vi "Adjust Magnetic Field_Continuous CW.vi"() -> ()   [LabVIEW 2020]
uses:
  Labview Library/Libraries/UT_Utilities/Utilities.lvlib
  Labview Library/Libraries/UT_Utilities/Support/Peak Parameter.ctl
  Labview Library/Libraries/Basic Experiment/Basic Experiment.lvlib
  Labview Library/Libraries/UT_Utilities/Support/Lorentizan Fit Parameter.ctl
  Labview Library/Libraries/Basic Experiment/CW settings.ctl
panel:
  in  "PS":string="X20.2 Y-0.4 Z16.5"
  in  "Theory Right Peak":dbl=1374.5
  in  "Calculate Right Peak":bool
  in  "Theory Left Peak":dbl=1374.5
  in  "Calculate Left Peak":bool
  in  "Add History":bool=TRUE
  in  "History":T2(array[cluster])
  in  "Zero Field Frequency":dbl=1360.0
  in  "Left Peak Settings":T3={"Num Pts"=20, "Start freq"=1205.0, "Stop freq"=1125.0, " dBm"=-10.0, "Loop times"=30000, "Ratio Thre(abs)"=0.03, "AutoTrace Before Exp"=FALSE, "RepoSave"=FALSE, "Peak Num Limit "=1}
  out "CW Left":cluster{"x":dbl[], "y":dbl[]}[](graph)=[{"x"=[1205.0, 1201.0, 1197.0, 1193.0, 1189.0, 1185.0, 1181.0, 1177.0, 1173.0, 1169.0, 1165.0, 1161.0, 1157.0, 1153.0, 1149.0, 1145.0, 1141.0, 1137.0, 1133.0, 1129.0, 1125.0], "y"=[-0.011159938681655596, -0.025153553670663936, -0.011876586772236327, 0.00021785543113589823, -0.012618639098234258, 0.004807904371223149, -0.00332547845045918, -0.001677185858675023, -0.0044172764590398005, -0.010320538540412821, -0.01357328707718994, -0.010368157455408136, -0.011699885854772149, -0.02274875266501088, -0.007152347209920283, -0.012399964822794828, -0.007602415395977236, -0.012597193866469744, -0.01720978929459495, -0.014711782800588472, -0.015376683926209849]}, {"x"=array[301 elements], "y"=[nan, nan, nan, nan, nan, nan, nan, nan, nan, nan, nan, nan, nan, nan, nan, nan, nan, nan, nan, nan, nan, nan, nan, nan, nan, nan, nan, nan, nan, nan, nan, nan, nan, nan, nan, nan, nan, nan, nan, nan, nan, nan, nan, nan, nan, nan, nan, nan, nan, nan, nan, nan, nan, nan, nan, nan, nan, nan, nan, nan, nan, nan, nan, nan, nan, nan, nan, nan, nan, nan, nan, nan, nan, nan, nan, nan, nan, nan, nan, nan, nan, nan, nan, nan, nan, nan, nan, nan, nan, nan, nan, nan, nan, nan, nan, nan, nan, nan, nan, nan, nan, nan, nan, nan, nan, nan, nan, nan, nan, nan, nan, nan, nan, nan, nan, nan, nan, nan, nan, nan, nan, nan, nan, nan, nan, nan, nan, nan, nan, nan, nan, nan, nan, nan, nan, nan, nan, nan, nan, nan, nan, nan, nan, nan, nan, nan, nan, nan, nan, nan, nan, nan, nan, nan, nan, nan, nan, nan, nan, nan, nan, nan, nan, nan, nan, nan, nan, nan, nan, nan, nan, nan, nan, nan, nan, nan, nan, nan, nan, nan, nan, nan, nan, nan, nan, nan, nan, nan, nan, nan, nan, nan, nan, nan, nan, nan, nan, nan, nan, nan, nan, nan, nan, nan, nan, nan, nan, nan, nan, nan, nan, nan, nan, nan, nan, nan, nan, nan, nan, nan, nan, nan, nan, nan, nan, nan, nan, nan, nan, nan, nan, nan, nan, nan, nan, nan, nan, nan, nan, nan, nan, nan, nan, nan, nan, nan, nan, nan, nan, nan, nan, nan, nan, nan, nan, nan, nan, nan, nan, nan, nan, nan, nan, nan, nan, nan, nan, nan, nan, nan, nan, nan, nan, nan, nan, nan, nan, nan, nan, nan, nan, nan, nan, nan, nan, nan, nan, nan, nan, nan, nan, nan, nan, nan, nan, nan, nan, nan, nan, nan, nan]}]
  in  "Left Fit Parameter":T4={"Background"=nan, "Peaks Parameter"=[]}
  in  "Right Fit Parameter":T4={"Background"=0.0056945852649640805, "Peaks Parameter"=[{"Amplitude"=-0.07797747065966305, "Position"=1532.2862299382655, "Width"=14.69533523973655}]}
  out "CW Right":cluster{"x":dbl[], "y":dbl[]}[](graph)=[{"x"=[1520.0, 1523.5, 1527.0, 1530.5, 1534.0, 1537.5, 1541.0, 1544.5, 1548.0, 1551.5, 1555.0, 1558.5, 1562.0, 1565.5, 1569.0, 1572.5, 1576.0, 1579.5, 1583.0, 1586.5, 1590.0], "y"=[-0.04503608389240439, -0.048468161356584064, -0.06917413643541893, -0.06935774109701642, -0.06266092515315635, -0.06993709008164904, -0.057095591522847176, -0.044065051622916525, -0.03324762033653629, -0.026683780314801054, -0.011314460872701045, 0.002465096474912041, -0.0038063202620164647, -0.005934718100890208, 0.0013360945954973612, 0.006420007158196134, -0.005723031875956611, -0.014175914235718875, -0.006224388082844169, 0.008040380578014025, -0.010785893304690297]}, {"x"=array[301 elements], "y"=array[301 elements]}]
  in  "Right Peak Settings":T3={"Num Pts"=20, "Start freq"=1520.0, "Stop freq"=1590.0, " dBm"=-13.0, "Loop times"=30000, "Ratio Thre(abs)"=0.04, "AutoTrace Before Exp"=FALSE, "RepoSave"=FALSE, "Peak Num Limit "=1}
  in  "Left Peak":bool
  in  "Right Peak":bool=TRUE
  in  "stop":bool
  in  "Enqueue Element":bool
  # "CW Settings"
  # "CW Settings"
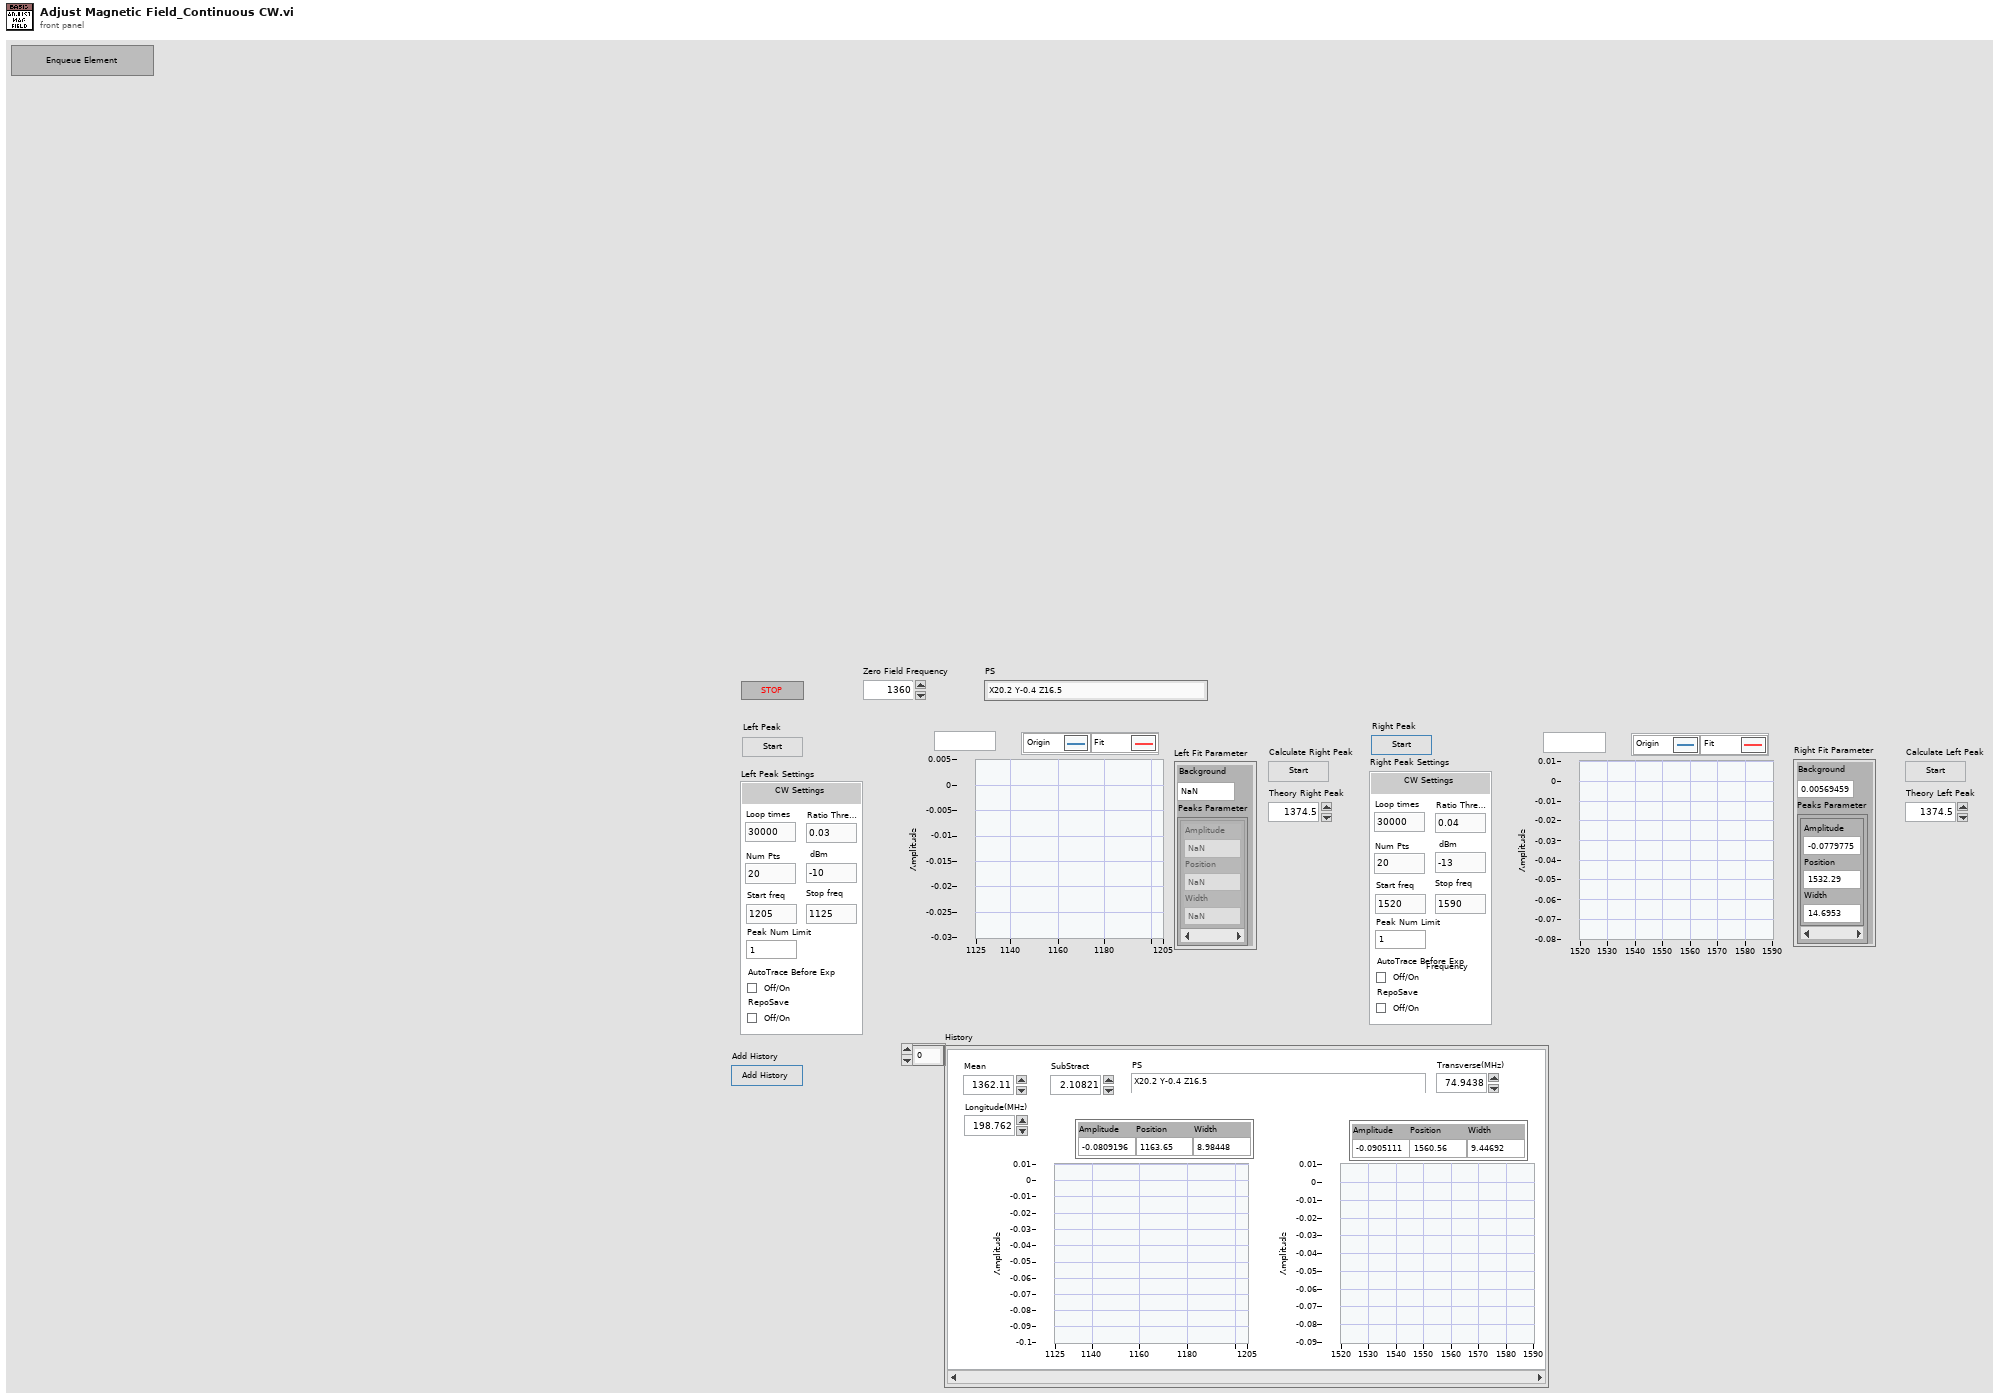
[diagram p1: front panel]
types:
  T1 = typedef "Utilities.lvlib/Peak Parameter.ctl" = cluster{"Amplitude":dbl, "Position":dbl, "Width":dbl}
  T2 = cluster{"Mean":dbl, "SubStract":dbl, "PS":string, "CW Left":cluster{"x":dbl[], "y":dbl[]}[], "CW Right":cluster{"x":dbl[], "y":dbl[]}[], "Left Peak Parameter":T1, "Right Peak Parameter":T1, "Longitude(MHz)":dbl, "Transverse(MHz)":dbl}[]
  T3 = typedef "Basic Experiment.lvlib/CW settings.ctl" = cluster{"Num Pts":i32, "Start freq":dbl, "Stop freq":dbl, " dBm":dbl, "Loop times":i32, "Ratio Thre(abs)":dbl, "AutoTrace Before Exp":bool, "RepoSave":bool, "Peak Num Limit ":i32}
  T4 = typedef "Utilities.lvlib/Lorentizan Fit Parameter.ctl" = cluster{"Background":dbl, "Peaks Parameter":T1[]}
  T5 = cluster{"Mean":dbl, "SubStract":dbl, "PS":string, "CW Left":cluster{"x":dbl[], "y":dbl[]}[], "CW Right":cluster{"x":dbl[], "y":dbl[]}[], "Left Peak Parameter":T1, "Right Peak Parameter":T1, "Longitude(MHz)":dbl, "Transverse(MHz)":dbl}
  T6 = typedef "Basic Experiment.lvlib/CW Results.ctl" = cluster{"Fit Frequency":T7, "Pro":dbl[], "Error Bar":dbl[], "Raw Data Path":path, "Image Path":path}
  T7 = typedef "Basic Experiment.lvlib/CW Fit Frequency.ctl" = cluster{"Fre2":cluster{"Amplitude":dbl, "Position":dbl, "Width":dbl}, "Fre1":cluster{"Amplitude":dbl, "Position":dbl, "Width":dbl}, "Fre3":cluster{"Amplitude":dbl, "Position":dbl, "Width":dbl}, "Background":dbl}
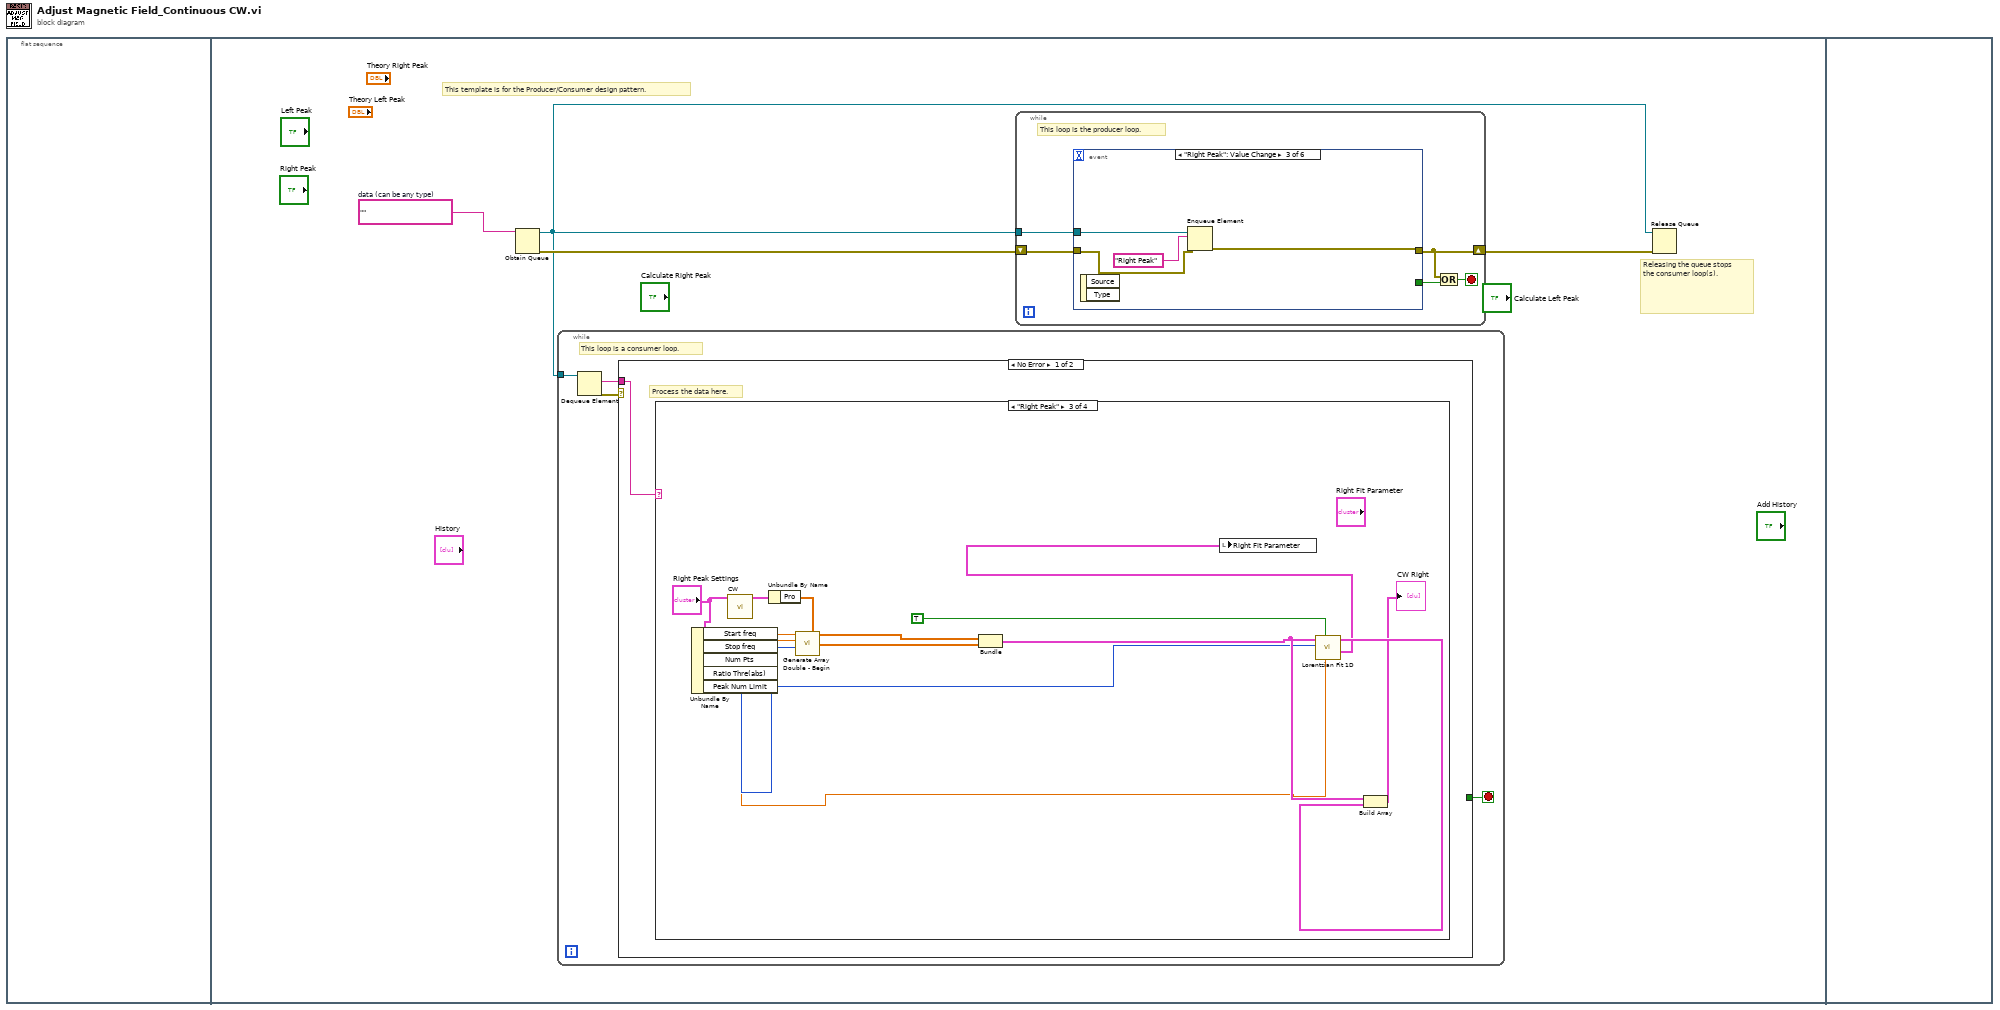
[diagram p0: block diagram]
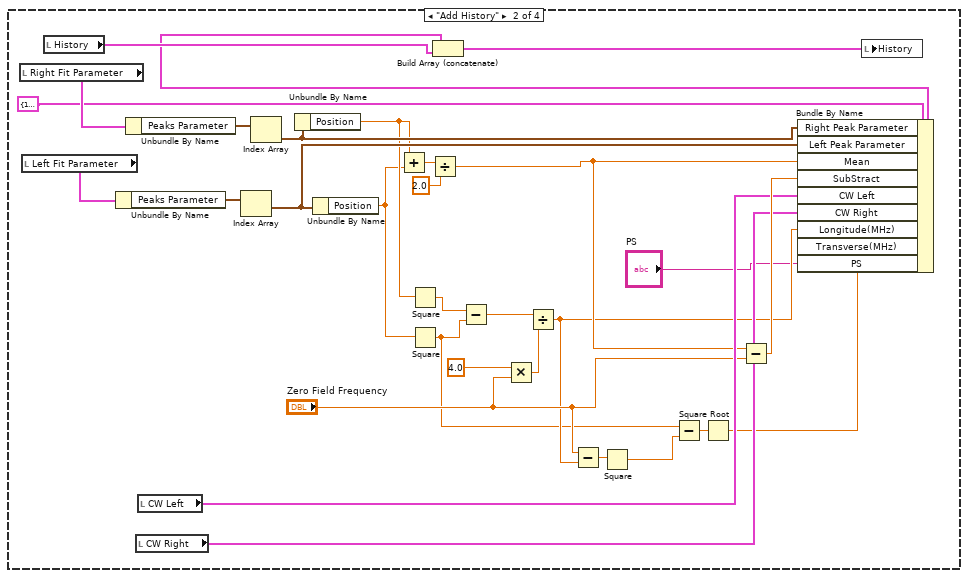
[diagram p3: hidden frame]
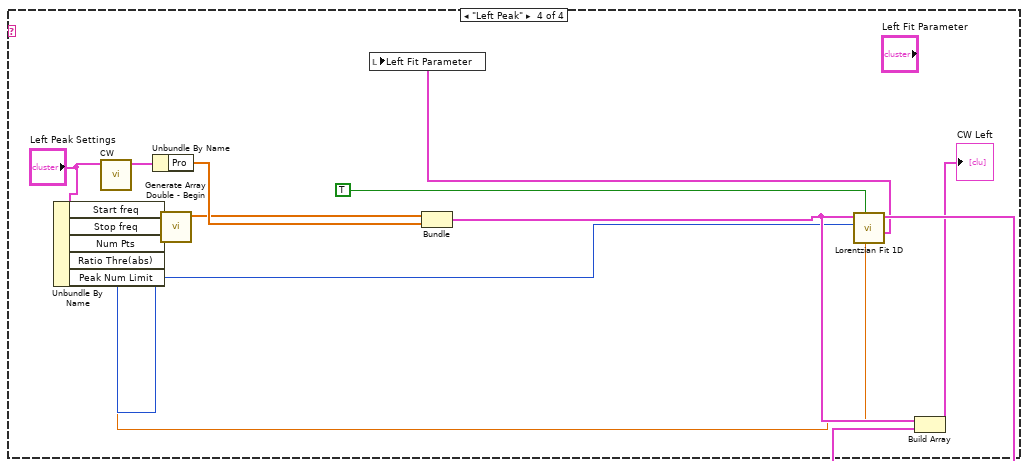
[diagram p4: hidden frame]
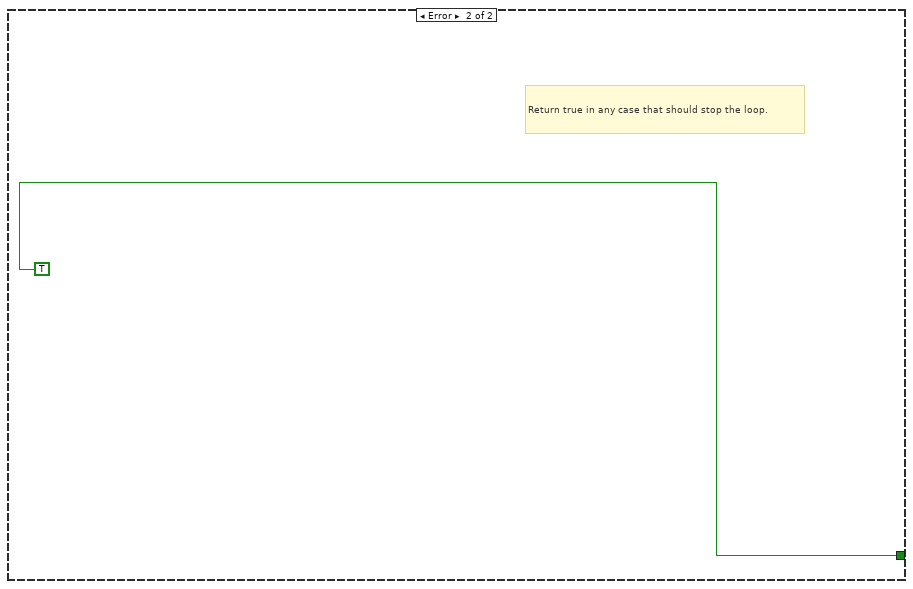
[diagram p5: hidden frame]
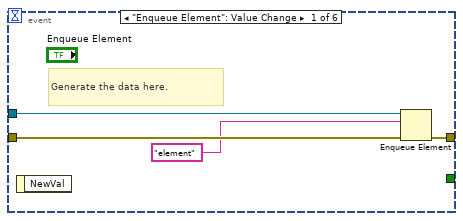
[diagram p6: hidden frame]
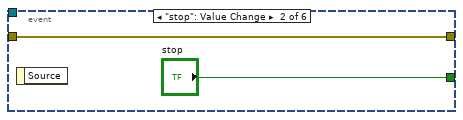
[diagram p7: hidden frame]
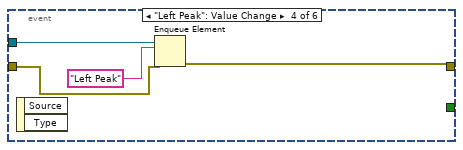
[diagram p8: hidden frame]
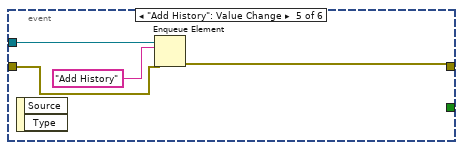
[diagram p9: hidden frame]
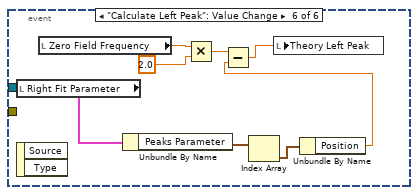
[diagram p10: hidden frame]
diagram:
  n1 = flat-sequence {
    frame #0 {
    }
    frame #1 {
      w2 = ""  # data (can be any type)
      # "Releasing the queue stops the consumer loop(s)."
      # "This template is for the Producer/Consumer design pattern."
      n2 = Obtain Queue(element data type=w2) -> (queue out=w1:refnum<queue>, error out=w4:errorcluster)  [unwired: 4 in, 1 out]
      n3 = while {
        tunnel: w1 -> [w8]
        stop <- w5 stop-if-true
        # "This loop is a consumer loop."
        n4 = Dequeue Element(queue=w8) -> (element=w6:string, error out=w7:errorcluster)  [unwired: 2 in, 2 out]
        n5 = case shown="No Error" w7 {
          tunnel: w6 -> [w9 _]
          tunnel: [_ TRUE] -> w5
          frame No Error {
            # "Process the data here."
            n6 = case shown="\"Right Peak\"" w9 {
              frame "False", Default {
              }
              frame "Add History" {
                n7 = local read "Right Fit Parameter"() -> (w36:T4)
                n8 = local read "Left Fit Parameter"() -> (w39:T4)
                n9 = local read "History"() -> (w31:T2)
                n10 = Unbundle By Name(w39) -> ("Peaks Parameter"=w38:T1[])
                n11 = Unbundle By Name(w36) -> ("Peaks Parameter"=w37:T1[])
                n12 = local read "CW Right"() -> (w28:cluster{"x":dbl[], "y":dbl[]}[])
                n13 = local read "CW Left"() -> (w29:cluster{"x":dbl[], "y":dbl[]}[])
                n14 = Index Array(array=w38) -> (element=w25:T1)  [unwired: 1 in]
                n15 = Index Array(array=w37) -> (element=w24:T1)  [unwired: 1 in]
                n16 = Unbundle By Name(w24) -> ("Position"=w23:dbl)
                n17 = Unbundle By Name(w25) -> ("Position"=w14:dbl)
                n18 = Add(x=w23, y=w14) -> (x+y=w35:dbl)
                n19 = Square(x=w23) -> (x^2=w22:dbl)
                n20 = Square(x=w14) -> (x^2=w11:dbl)
                n21 = Divide(x=w35, y=2.0) -> (x/y=w26:dbl)
                n22 = Subtract(x=w22, y=w11) -> (x-y=w21:dbl)
                n23 = Multiply(x=4.0, y="Zero Field Frequency") -> (x*y=w19:dbl)
                n24 = Divide(x=w21, y=w19) -> (x/y=w17:dbl)
                n25 = Subtract(x="Zero Field Frequency", y=w17) -> (x-y=w16:dbl)
                n26 = Square(x=w16) -> (x^2=w15:dbl)
                n27 = Subtract(x=w11, y=w15) -> (x-y=w13:dbl)
                n28 = Square Root(x=w13) -> (sqrt(x)=w12:dbl)
                n29 = Subtract(x=w26, y="Zero Field Frequency") -> (x-y=w33:dbl)
                n30 = Bundle By Name(cluster=T5 {"Mean"=1414.1094924647537, "SubStract"=39.60949246475366, "PS"="", "CW Left"=[], "CW Right"=[], "Left Peak Parameter"={"Amplitude"=-0.05552543645018247, "Position"=1349.4629709624935, "Width"=6.25}, "Right Peak Parameter"={"Amplitude"=-0.09115089462235382, "Position"=1478.7560139670136, "Width"=6.817754325190208}, "Longitude(MHz)"=nan, "Transverse(MHz)"=nan} ("History"), "Right Peak Parameter"=w24, "Left Peak Parameter"=w25, "Mean"=w26, "SubStract"=w33, "CW Left"=w29, "CW Right"=w28, "Longitude(MHz)"=w17, "Transverse(MHz)"=w12, "PS"="PS") -> (w30:T5)
                n31 = Build Array (concatenate)(w30, w31) -> (w32:T2)
                n32 = local write "History"(w32) -> ()
              }
              frame "Right Peak" {
                n33 = Unbundle By Name("Right Peak Settings") -> ("Start freq"=w49:dbl, "Stop freq"=w48:dbl, "Num Pts"=w47:i32, "Ratio Thre(abs)"=w42:dbl, "Peak Num Limit"=w40:i32)
                n34 = call "CW.vi"("Settings"="Right Peak Settings") -> ("CW Result"=w51:T6)  [unwired: 8 in, 2 out]
                n35 = Unbundle By Name(w51) -> ("Pro"=w50:dbl[])
                n36 = call "Generate Array Double - Begin.vi"("num of step"=w47, "end"=w48, "begin"=w49) -> ("output array"=w45:dbl[])  [unwired: 5 in, 3 out]
                n37 = Bundle("output array"=w45, "Pro"=w50) -> (w44:cluster{"output array":dbl[], "Pro":dbl[]})  [unwired: 1 in]
                n38 = call "Lorentzian Fit 1D.vi"("Amplitude Limit (0.05)"=w42, "Reverse Peak?"=TRUE, "Peak Number Limit (10)"=w40, "Data"=w44) -> ("Best Fit Parameter"=w41:T4, "Fit Result"=w53:cluster{"x":dbl[], "y":dbl[]})  [unwired: 3 in, 3 out]
                n39 = local write "Right Fit Parameter"(w41) -> ()
                n40 = Build Array(w44, w53) -> (→"CW Right":cluster{"x":dbl[], "y":dbl[]}[])
              }
              frame "Left Peak" {
                n41 = Unbundle By Name("Left Peak Settings") -> ("Start freq"=w63:dbl, "Stop freq"=w62:dbl, "Num Pts"=w61:i32, "Ratio Thre(abs)"=w56:dbl, "Peak Num Limit"=w54:i32)
                n42 = call "CW.vi"("Settings"="Left Peak Settings") -> ("CW Result"=w65:T6)  [unwired: 8 in, 2 out]
                n43 = Unbundle By Name(w65) -> ("Pro"=w64:dbl[])
                n44 = call "Generate Array Double - Begin.vi"("num of step"=w61, "end"=w62, "begin"=w63) -> ("output array"=w59:dbl[])  [unwired: 5 in, 3 out]
                n45 = Bundle("output array"=w59, "Pro"=w64) -> (w58:cluster{"output array":dbl[], "Pro":dbl[]})  [unwired: 1 in]
                n46 = call "Lorentzian Fit 1D.vi"("Amplitude Limit (0.05)"=w56, "Reverse Peak?"=TRUE, "Peak Number Limit (10)"=w54, "Data"=w58) -> ("Best Fit Parameter"=w55:T4, "Fit Result"=w67:cluster{"x":dbl[], "y":dbl[]})  [unwired: 3 in, 3 out]
                n47 = local write "Left Fit Parameter"(w55) -> ()
                n48 = Build Array(w58, w67) -> (→"CW Left":cluster{"x":dbl[], "y":dbl[]}[])
              }
            }
          }
          frame Error {
            # "Return true in any case that should stop the loop."
          }
        }
      }
      n49 = while {
        shift-right: [w69] -> w3
        shift-left: w4 -> [w72]
        tunnel: w1 -> [w73]
        stop <- w70 stop-if-true
        # "This loop is the producer loop."
        n50 = event shown="[2] \"Right Peak\": Value Change" {
          selector: _ -> [_ _ _ _ _ _]
          dyn-events: _ -> [_ _ _ _ _ _]
          timeout: _ -> [_ _ _ _ _ _]
          tunnel: w73 -> [w77 _ w82 w86 w90 _]
          tunnel: w72 -> [w76 w78 w81 w85 w89 _]
          tunnel: [w75 w78 w80 w84 w88 _] -> w69
          tunnel: [_ "stop" _ _ _ _] -> w71
          event "Enqueue Element": Value Change {
            # "Generate the data here."
            n51 = event-data() -> ()  [unwired: 1 in, 1 out]
            n52 = Enqueue Element(queue=w77, element="element", error in (no error)=w76) -> (error out=w75:errorcluster)  [unwired: 1 in, 2 out]
          }
          event "stop": Value Change {
            n53 = event-data() -> ()  [unwired: 1 in, 1 out]
          }
          event "Right Peak": Value Change {
            n54 = event-data() -> ()  [unwired: 1 in, 2 out]
            n55 = Enqueue Element(queue=w82, element="Right Peak", error in (no error)=w81) -> (error out=w80:errorcluster)  [unwired: 1 in, 2 out]
          }
          event "Left Peak": Value Change {
            n56 = event-data() -> ()  [unwired: 1 in, 2 out]
            n57 = Enqueue Element(queue=w86, element="Left Peak", error in (no error)=w85) -> (error out=w84:errorcluster)  [unwired: 1 in, 2 out]
          }
          event "Add History": Value Change {
            n58 = event-data() -> ()  [unwired: 1 in, 2 out]
            n59 = Enqueue Element(queue=w90, element="Add History", error in (no error)=w89) -> (error out=w88:errorcluster)  [unwired: 1 in, 2 out]
          }
          event "Calculate Left Peak": Value Change {
            n60 = local read "Right Fit Parameter"() -> (w95:T4)
            n61 = event-data() -> ()  [unwired: 1 in, 2 out]
            n62 = local read "Zero Field Frequency"() -> (w99:dbl)
            n63 = Unbundle By Name(w95) -> ("Peaks Parameter"=w96:T1[])
            n64 = Multiply(x=w99, y=2.0) -> (x*y=w97:dbl)
            n65 = Index Array(array=w96) -> (element=w94:T1)  [unwired: 1 in]
            n66 = Unbundle By Name(w94) -> ("Position"=w93:dbl)
            n67 = Subtract(x=w97, y=w93) -> (x-y=w92:dbl)
            n68 = local write "Theory Left Peak"(w92) -> ()
          }
        }
        n69 = Or(x=w69, y=w71) -> (x .or. y?=w70:bool)
      }
      n70 = Release Queue(queue=w1, error in (no error)=w3) -> ()  [unwired: 1 in, 3 out]
    }
    frame #2 {
    }
  }
